vi "get_run_mode.vi"(8 "error in (no error)":errorcluster, 11 "GenericPlugin in":refnum<class "GenericComponent.lvclass">) -> (0 "error out":errorcluster, 2 "run mode":T1=enum."single sweep mode", 3 "GenericPlugin out":refnum<class "GenericComponent.lvclass">, 4 "is NOT free run?":bool, 6 "is free run?":bool)   [LabVIEW 2010, in "GenericComponent.lvclass"]
uses:
  GenericComponent.lvclass
  main/labview_source/type_definitions/enumerations/run_mode_enum.ctl
  class_data.vi
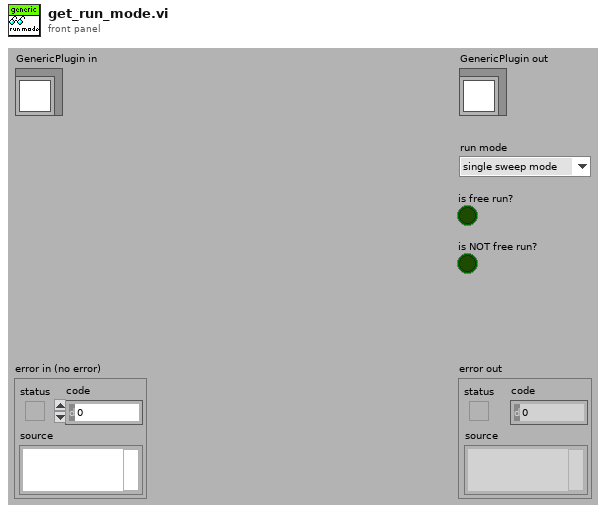
[diagram p1: front panel]
types:
  T1 = typedef "run_mode_enum.ctl" = enum16{"focus mode", "single sweep mode", "experiment mode"}
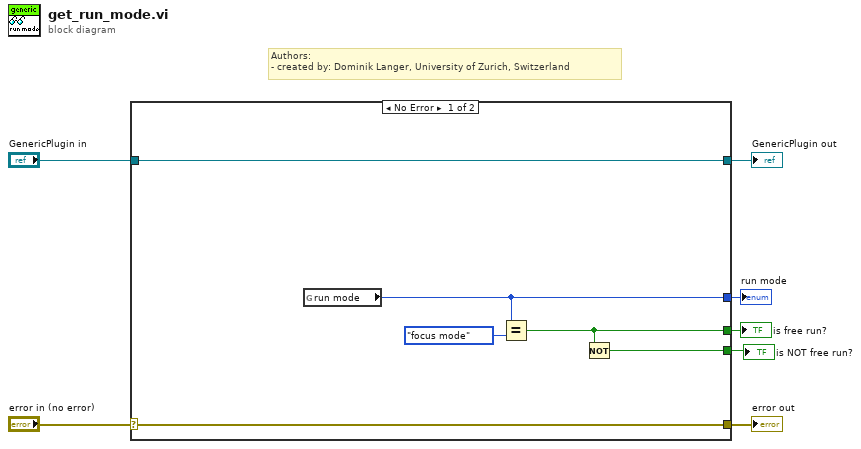
[diagram p0: block diagram]
diagram:
  # "Authors: \n- created by: Dominik Langer, University of Zurich, Switzerland"
  n1 = case shown="No Error" "error in (no error)" {
    selector: "error in (no error)" -> [w12 w15]
    tunnel: [w12 w15] -> w6
    tunnel: [w13 w14] -> w4
    tunnel: "GenericPlugin in" -> [w13 w14]
    tunnel: [w11 _] -> w3
    tunnel: [w9 _] -> w2
    tunnel: [w8 _] -> w1
    frame No Error {
      n2 = global read "class_data.vi" "run mode"() -> (w11:T1)
      n3 = Equal?(x=w11, y=run_mode_enum."focus mode") -> (x = y?=w9:bool)
      n4 = Not(x=w9) -> (.not. x?=w8:bool)
    }
    frame Error {
    }
  }
  "error out" <- w6
  "GenericPlugin out" <- w4
  "run mode" <- w3
  "is free run?" <- w2
  "is NOT free run?" <- w1
